vi "Read Clock.vi"(8 "error in (no error)":errorcluster, 11 "VISA resource name":refnum<visa-resource-name>) -> (0 "error out":errorcluster, 2 "Clock Reading":string, 3 "VISA resource name out":refnum<visa-resource-name>)   [LabVIEW 2016, in "EFD Ultimus V.lvlib"]
doc: "Reads the time from the real time clock on the Ultimus V. 'D0' is the letter 'D' followed by the digit '0'.\n\nHost Format: EE--\n\nReturn Format:D0HhhMmmAMa\nhh:Hours 0-23 for 24 hour format, 1-12 for 12 hour format\nmm: Minutes 0-59\na:Hour format 0=AM,1=PM,2=24 Hour Format"
uses:
  EFD Ultimus V.lvlib
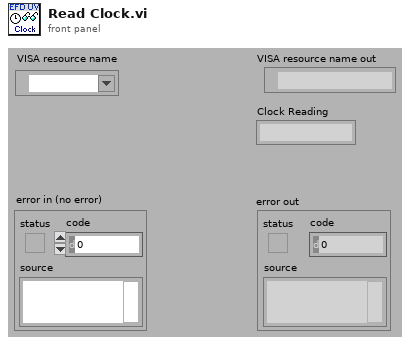
[diagram p1: front panel]
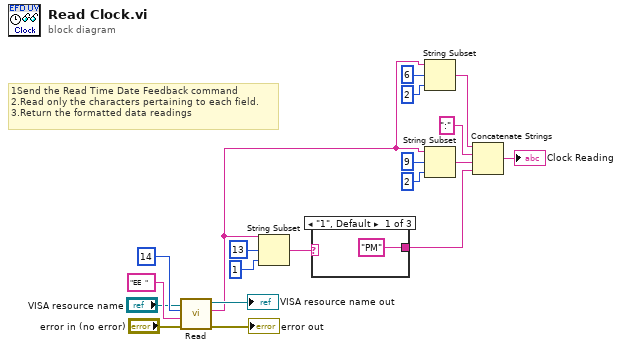
[diagram p0: block diagram]
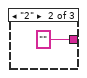
[diagram p2: hidden frame]
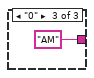
[diagram p3: hidden frame]
diagram:
  # "1Send the Read Time Date Feedback command\n2.Read only the characters pertaining to each field.\n3.Return the formatted data readings"
  n1 = call "Read.vi"("error in (no error)"="error in (no error)", "Command To Write"="EE  ", "Bytes to Read (11)"=u32 14 ("Bytes to Read from Buffer"), "VISA resource name"="VISA resource name") -> ("error out"=→"error out":errorcluster, "Ultimus V Feedback Data"=w8:string, "VISA resource name out"=→"VISA resource name out":refnum<visa-resource-name>)  [unwired: 5 in]
  n2 = String Subset(string=w8, offset (0)=13, length (rest)=1 ("length (rest)")) -> (substring=w19:string)
  n3 = case shown="\"1\", Default" w19 {
    tunnel: ["PM" "" "AM"] -> w3
    frame "1", Default {
    }
    frame "2" {
    }
    frame "0" {
    }
  }
  n4 = String Subset(string=w8, offset (0)=6, length (rest)=2 ("length (rest)")) -> (substring=w6:string)
  n5 = String Subset(string=w8, offset (0)=9, length (rest)=2 ("length (rest)")) -> (substring=w5:string)
  n6 = Concatenate Strings(w6, ":" ("string"), w5, w3) -> (→"Clock Reading":string)
